vi "2 ^ n Gain.vi"(1 "18b (s-fxp-1) in":fxp<+/-,18,1> format="%.18g", 2 "N":i8) -> (0 "18b (s-fxp-1) out":fxp<+/-,18,1> format="%.18g")   [LabVIEW 2009]
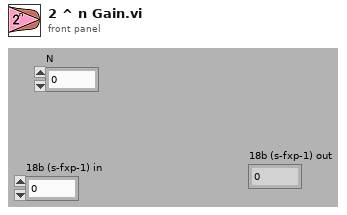
[diagram p1: front panel]
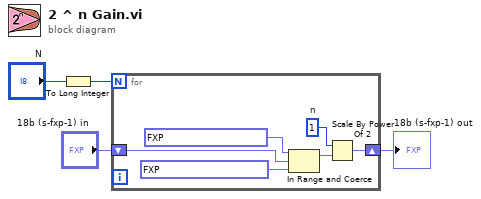
[diagram p0: block diagram]
diagram:
  n1 = To Long Integer(number="N") -> (32bit integer=w1:i32)
  n2 = for {
    N: w1 -> [_]
    shift-right: [w7] -> w2
    shift-left: "18b (s-fxp-1) in" -> [w9]
    w10 = 1  # n
    n3 = In Range and Coerce(upper limit=fxp<+/-,18,1> 0.4999847412109375, x=w9, lower limit=fxp<+/-,18,1> -0.5) -> (coerced(x)=w8:fxp<+/-,18,1>)  [unwired: 1 out]
    n4 = Scale By Power Of 2(n=w10, x=w8) -> (x*2^n=w7:fxp<+/-,18,1>)
  }
  "18b (s-fxp-1) out" <- w2
